vi "RPI.SenseHat Init.vi"(8 "error in (no error)":errorcluster, 11 "RPI.SenseHat.Actor in":refnum<class "RPI.SenseHat.Actor.lvclass">) -> (0 "error out":errorcluster, 3 "RPI.SenseHat.Actor out":refnum<class "RPI.SenseHat.Actor.lvclass">)   [LabVIEW 2020, in "RPI.SenseHat.Actor.lvlib" / "RPI.SenseHat.Actor.lvclass"]
uses:
  RPI.SenseHat.Actor.lvclass
  RPI.SenseHat.Actor.lvclass/RPI.SenseHat.Actor.ctl
  <vilib>/MakerHub/LINX/Public/Utilities/Open Local.vi
  RPI.SenseHat/SenseHat/SenseHat.lvclass
  <vilib>/MakerHub/LINX/LMH-LINX.lvlib
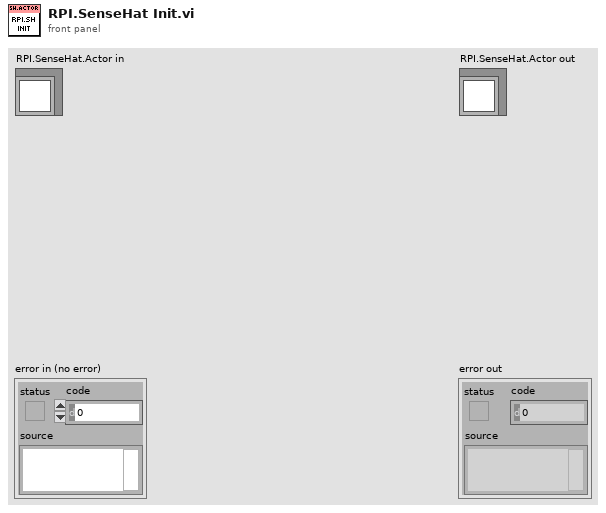
[diagram p1: front panel]
types:
  T1 = typedef "LMH-LINX.lvlib/LINX Ref.ctl" = cluster{"IO":T2, "Interface":T3, "LINX Device Config":T4}
  T2 = typedef "LMH-LINX.lvlib/Platform.ctl" = enum16{"Remote", "Local"}
  T3 = typedef "LMH-LINX.lvlib/Interface.ctl" = enum16{"Serial", "TCP"}
  T4 = typedef "LMH-LINX.lvlib/Device.lvlib/LINX Device Config.ctl" = cluster{"Interface":T3, "COM Port":refnum<visa-resource-name>, "TCP Configuration":T5, "Device Family":u8, "Device ID":u8, "Device Name":string, "TCP Ref":refnum<k5>, "Channels":T6}
  T5 = typedef "LMH-LINX.lvlib/Device.lvlib/TCP Config.ctl" = cluster{"IP Address":string, "Port":u16}
  T6 = typedef "LMH-LINX.lvlib/Channels.ctl" = cluster{"DI":u8[], "DO":u8[], "AI":u8[], "AO":u8[], "PWM":u8[], "QE":u8[], "UART":u8[], "I2C 2":u8[], "SPI":u8[], "CAN":u8[], "Servo":u8[], "AI Ref (V)":dbl, "AI Resolution (Bits)":u8, "AO Ref (V)":dbl, "AO Resolution (Bits)":u8}
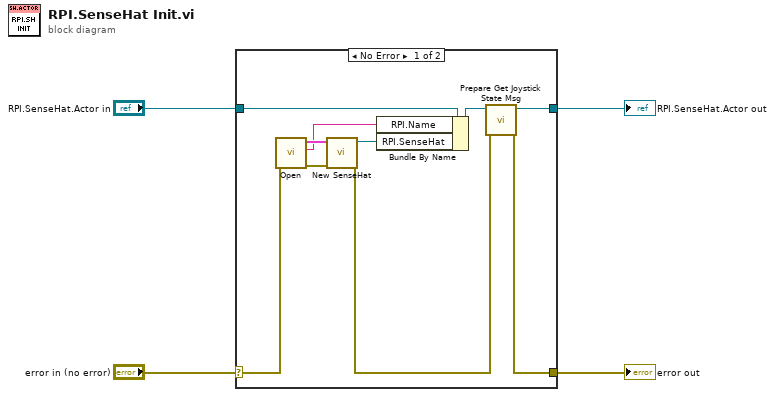
[diagram p0: block diagram]
diagram:
  n1 = case shown="No Error" "error in (no error)" {
    selector: "error in (no error)" -> [w9 w16]
    tunnel: [w5 w16] -> w3
    tunnel: [w7 w15] -> w1
    tunnel: "RPI.SenseHat.Actor in" -> [w14 w15]
    frame No Error {
      n2 = call-poly <vilib>:"Open.vi"("Error In"=w9) -> ("Error Out"=w12:errorcluster, "Device Name"=w11:string, "LINX Resource"=w13:T1)  [unwired: 8 in]
      n3 = call "New SenseHat.vi"("error in (no error)"=w12, "LINX Resource"=w13) -> ("error out"=w6:errorcluster, "SenseHat out"=w10:refnum<class "SenseHat.lvclass">)  [unwired: 8 in]
      n4 = Bundle By Name(cluster=w14, "RPI.Name"=w11, "RPI.SenseHat"=w10) -> (w8:refnum<class "RPI.SenseHat.Actor.lvclass">)
      n5 = call "Prepare Get Joystick State Msg.vi"("error in (no error)"=w6, "RPI.SenseHat.Actor in"=w8) -> ("error out"=w5:errorcluster, "RPI.SenseHat.Actor out"=w7:refnum<class "RPI.SenseHat.Actor.lvclass">)  [unwired: 8 in]
    }
    frame Error {
    }
  }
  "error out" <- w3
  "RPI.SenseHat.Actor out" <- w1
